vi "Write Key I16.vi"(7 "Section Name":string, 8 "error in":errorcluster, 9 "New Value":i16, 10 "Key Name":string, 11 "Config Cluster in":T1) -> (0 "error out":errorcluster, 3 "Config File.lvclass out":T1)   [LabVIEW 2017]
uses:
  Config Cluster.ctl
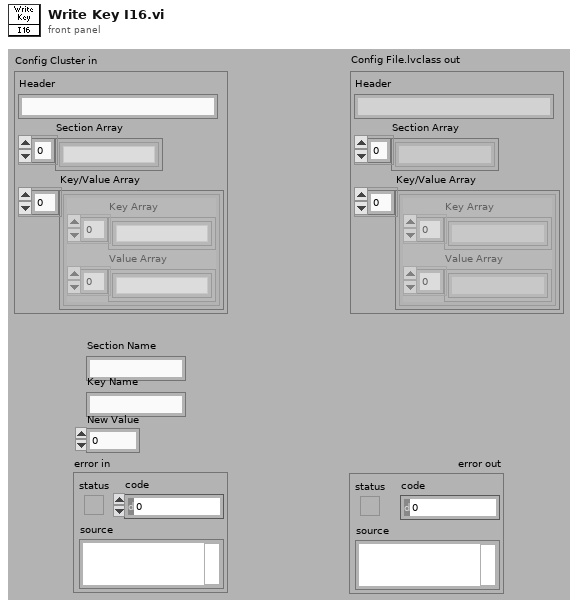
[diagram p1: front panel]
types:
  T1 = typedef "Config Cluster.ctl" = cluster{"Header":string, "Section Array":string[], "Key/Value Array":cluster{"Key Array":string[], "Value Array":string[]}[]}
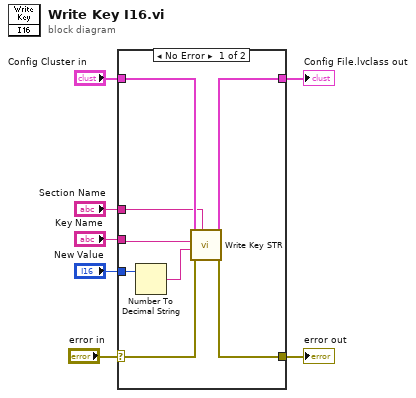
[diagram p0: block diagram]
diagram:
  n1 = case shown="No Error" "error in" {
    selector: "error in" -> [w13 w16]
    tunnel: [w12 w16] -> w6
    tunnel: "Config Cluster in" -> [w10 w17]
    tunnel: [w11 w17] -> w4
    tunnel: "Section Name" -> [w9 _]
    tunnel: "Key Name" -> [w8 _]
    tunnel: "New Value" -> [w15 _]
    frame No Error {
      n2 = Number To Decimal String(number=w15) -> (decimal integer string=w14:string)  [unwired: 1 in]
      n3 = call "Write Key STR.vi"("Section Name"=w9, "error in"=w13, "New Value"=w14, "Key Name"=w8, "Config Cluster in"=w10) -> ("error out"=w12:errorcluster, "Config Cluster out"=w11:T1)  [unwired: 5 in]
    }
    frame Error {
    }
  }
  "error out" <- w6
  "Config File.lvclass out" <- w4
